vi "get from nxt.vi"() -> ()   [LabVIEW 2011, in "talk.lvrbt"]
uses:
  talk.lvrbt
  <vilib>/NXT/Block Support/NXT_MessageMailbox.ctl
  <vilib>/NXT/Dual Mode Library/BT/BlueTooth_Read_num.vi
panel:
  out "Message":i32
  out "Blink":bool
  in  "stop":bool
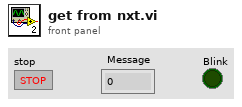
[diagram p1: front panel]
types:
  T1 = typedef "NXT_MessageMailbox.ctl" = u8
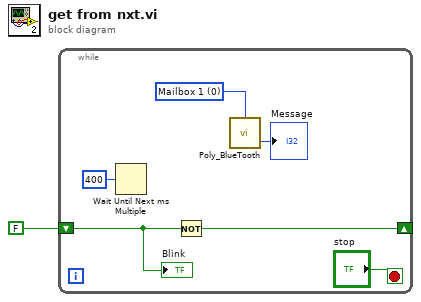
[diagram p0: block diagram]
diagram:
  n1 = while {
    shift-right: [w4] -> _
    shift-left: FALSE -> [w5]
    stop <- "stop" stop-if-true
    w3 = T1 0 items=["Mailbox 1", "Mailbox 2", "Mailbox 3", "Mailbox 4", "Mailbox 5", "Mailbox 6", "Mailbox 7", "Mailbox 8", "Mailbox 9", "Mailbox 10"] ("Mailbox")
    n2 = Wait Until Next ms Multiple(millisecond multiple=u32 400) -> ()  [unwired: 1 out]
    n3 = Not(x=w5) -> (.not. x?=w4:bool)
    n4 = call-poly <vilib>:"Poly_BlueTooth.vi"("Mailbox"=w3) -> ("Message"=→"Message":i32)  [unwired: 2 in, 1 out]
    "Blink" <- w5
  }
